vi "Read XML_Parse BC.vi"(8 "error in (no error)":errorcluster, 10 "channel":T1, 11 ".NET Refnum in":refnum<k24>) -> (0 "error out":errorcluster, 2 "channel out":T1, 3 ".NET Refnum out":refnum<k24>)   [LabVIEW 2017, in "Ballard 1553 System Explorer.lvlib"]
uses:
  Ballard 1553 System Explorer.lvlib
  Ballard_Channel.ctl
  Ballard_BC.ctl
  Ballard_message.ctl
  Ballard_messageType.ctl
  Ballard_CWD1.ctl
  Ballard_CWD2.ctl
  Ballard_minorFrame.ctl
  Ballard_majorFrame.ctl
  Ballard_acyclicFrame.ctl
  Ballard_RT.ctl
  Ballard_RT subAddress.ctl
  Ballard_RT direction.ctl
  Ballard_RT rtMode.ctl
  Ballard_RT modeCode.ctl
  D:/Ballard-1553-Custom-Device Inline Async/Source/System Explorer/SubVIs/Parse XML Ballard/Ballard_BTI_XML_MIL_STD_1553_Deserializer.dll
  Ballard_BTI_XML_MIL_STD_1553_Deserializer.dll
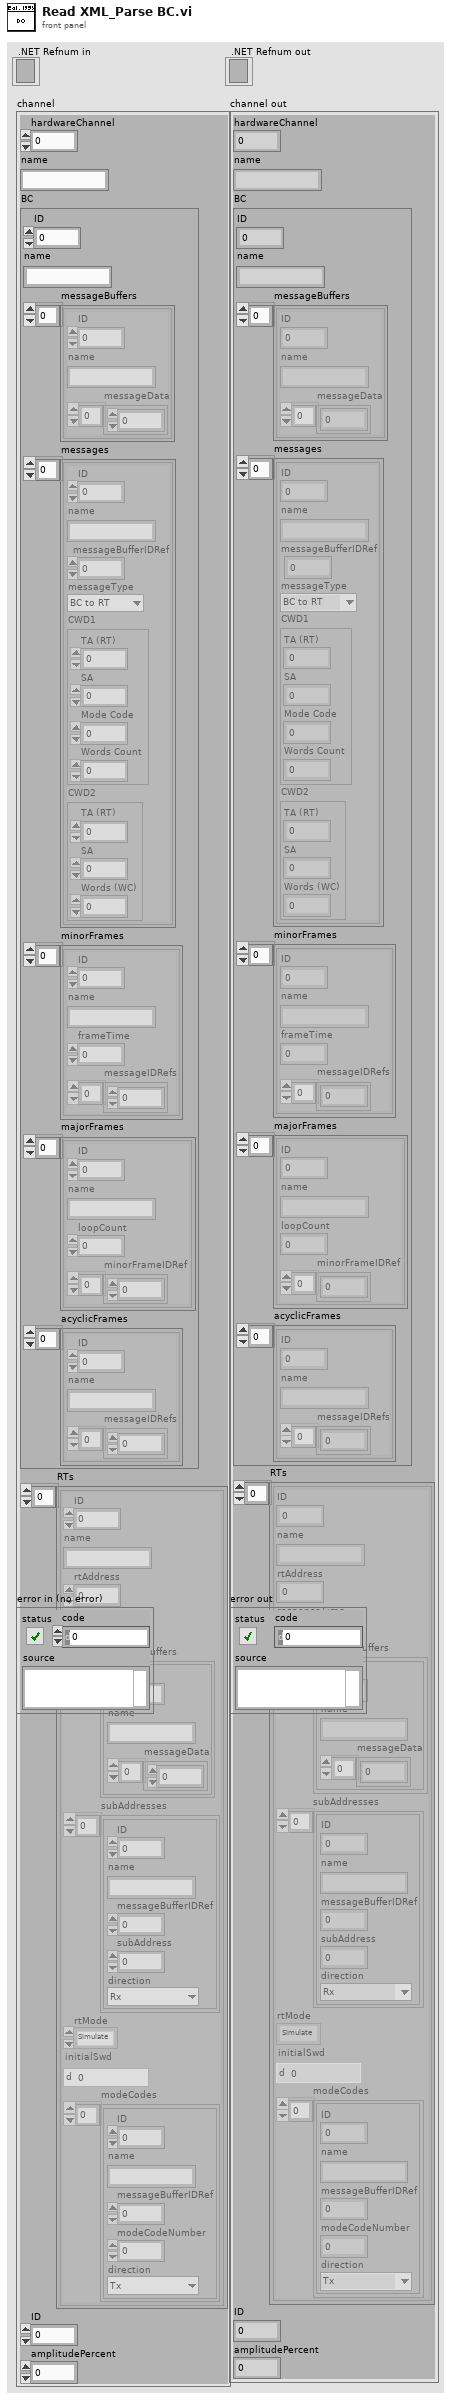
[diagram p1: front panel]
types:
  T1 = typedef "Ballard 1553 System Explorer.lvlib/Ballard_Channel.ctl" = cluster{"hardwareChannel":i32, "name":string, "BC":T2, "RTs":T10[], "ID":i32, "amplitudePercent":dbl}
  T2 = typedef "Ballard 1553 System Explorer.lvlib/Ballard_BC.ctl" = cluster{"ID":i32, "name":string, "messageBuffers":cluster{"ID":i32, "name":string, "messageData":u16[]}[], "messages":T3[], "minorFrames":T7[], "majorFrames":T8[], "acyclicFrames":T9[]}
  T3 = typedef "Ballard 1553 System Explorer.lvlib/Ballard_message.ctl" = cluster{"ID":i32, "name":string, "messageBufferIDRef":i32, "messageType":T4, "CWD1":T5, "CWD2":T6}
  T4 = typedef "Ballard 1553 System Explorer.lvlib/Ballard_messageType.ctl" = enum16{"BC to RT", "RT to BC", "RT to RT", "MC (Rx)", "MC (Tx)"}
  T5 = typedef "Ballard 1553 System Explorer.lvlib/Ballard_CWD1.ctl" = cluster{"TA (RT)":i8, "SA":i8, "Mode Code":i8, "Words Count":i8}
  T6 = typedef "Ballard 1553 System Explorer.lvlib/Ballard_CWD2.ctl" = cluster{"TA (RT)":i8, "SA":i8, "Words (WC)":i8}
  T7 = typedef "Ballard 1553 System Explorer.lvlib/Ballard_minorFrame.ctl" = cluster{"ID":i32, "name":string, "frameTime":i32, "messageIDRefs":i32[]}
  T8 = typedef "Ballard 1553 System Explorer.lvlib/Ballard_majorFrame.ctl" = cluster{"ID":i32, "name":string, "loopCount":i32, "minorFrameIDRef":i32[]}
  T9 = typedef "Ballard 1553 System Explorer.lvlib/Ballard_acyclicFrame.ctl" = cluster{"ID":i32, "name":string, "messageIDRefs":i32[]}
  T10 = typedef "Ballard 1553 System Explorer.lvlib/Ballard_RT.ctl" = cluster{"ID":i32, "name":string, "rtAddress":i8, "responseTime":i32, "messageBuffers":cluster{"ID":i32, "name":string, "messageData":u16[]}[], "subAddresses":T11[], "rtMode":T13, "initialSwd":u16, "modeCodes":T14[]}
  T11 = typedef "Ballard 1553 System Explorer.lvlib/Ballard_RT subAddress.ctl" = cluster{"ID":i32, "name":string, "messageBufferIDRef":i32, "subAddress":i8, "direction":T12}
  T12 = typedef "Ballard 1553 System Explorer.lvlib/Ballard_RT direction.ctl" = enum16{"Tx", "Rx"}
  T13 = typedef "Ballard 1553 System Explorer.lvlib/Ballard_RT rtMode.ctl" = enum16{"Simulate", "Monitor", "Disable"}
  T14 = typedef "Ballard 1553 System Explorer.lvlib/Ballard_RT modeCode.ctl" = cluster{"ID":i32, "name":string, "messageBufferIDRef":i32, "modeCodeNumber":i8, "direction":T12}
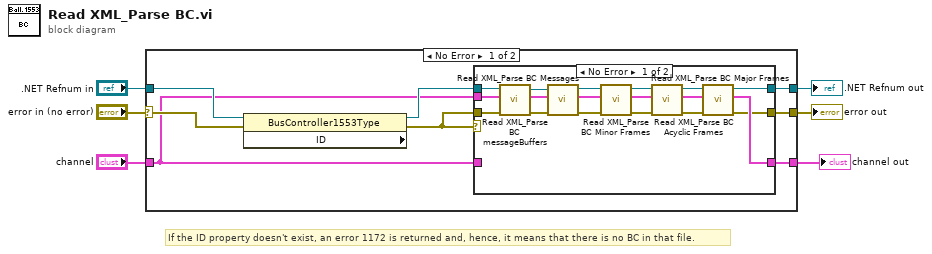
[diagram p0: block diagram]
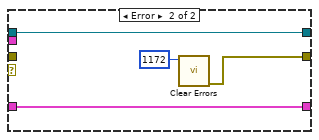
[diagram p2: hidden frame]
diagram:
  # "If the ID property doesn't exist, an error 1172 is returned and, hence, it means that there is no BC in that file."
  n1 = case shown="No Error" "error in (no error)" {
    selector: "error in (no error)" -> [w10 w38]
    tunnel: [w14 w37] -> w6
    tunnel: [w13 w39] -> w5
    tunnel: [w12 w38] -> w4
    tunnel: "channel" -> [w7 w37]
    tunnel: ".NET Refnum in" -> [w11 w39]
    frame No Error {
      n2 = property class="BusController1553Type" props=["ID"](reference=w11, error in=w10) -> (reference out=w9:refnum<k24>, error out=w8:errorcluster)  [unwired: 1 out]
      n3 = case shown="No Error" w8 {
        tunnel: w7 -> [w25 _]
        tunnel: [w19 w33] -> w14
        tunnel: [w18 w36] -> w13
        tunnel: [w17 w34] -> w12
        tunnel: w9 -> [w16 w36]
        tunnel: w8 -> [w15 _]
        tunnel: w7 -> [_ w33]
        frame No Error {
          n4 = call "Read XML_Parse BC messageBuffers.vi"("error in (no error)"=w15, "channel in"=w25, "BusController1553Type"=w16) -> ("error out"=w24:errorcluster, "channel out"=w26:T1, "BusController1553Type"=w23:refnum<k24>)  [unwired: 6 in]
          n5 = call "Read XML_Parse BC Messages.vi"("error in (no error)"=w24, "channel in"=w26, "BusController1553Type"=w23) -> ("error out"=w27:errorcluster, "channel out"=w29:T1, "BusController1553Type"=w28:refnum<k24>)  [unwired: 6 in]
          n6 = call "Read XML_Parse BC Minor Frames.vi"("error in (no error)"=w27, "channel in"=w29, "BusController1553Type"=w28) -> ("error out"=w31:errorcluster, "channel out"=w32:T1, "BusController1553Type"=w30:refnum<k24>)  [unwired: 6 in]
          n7 = call "Read XML_Parse BC Major Frames.vi"("error in (no error)"=w31, "channel in"=w32, "BusController1553Type"=w30) -> ("error out"=w21:errorcluster, "channel out"=w20:T1, "BusController1553Type"=w22:refnum<k24>)  [unwired: 6 in]
          n8 = call "Read XML_Parse BC Acyclic Frames.vi"("error in (no error)"=w21, "channel in"=w20, "BusController1553Type"=w22) -> ("error out"=w17:errorcluster, "channel out"=w19:T1, "BusController1553Type"=w18:refnum<k24>)  [unwired: 6 in]
        }
        frame Error {
          n9 = call <vilib>:"Clear Errors.vi"("specific error code to clear (0: all)"=1172) -> ("error out"=w34:errorcluster)  [unwired: 5 in, 1 out]
        }
      }
    }
    frame Error {
    }
  }
  "channel out" <- w6
  ".NET Refnum out" <- w5
  "error out" <- w4
